vi "AutoCollectBall.vi"(8 "error in (no error)":errorcluster, 10 "PreCollectWait":u32=400, 11 "IsTwoBall?":bool) -> (0 "error out":errorcluster)   [LabVIEW 2013]
uses:
  DoubleSolenoidAction.ctl
  RollerAction.ctl
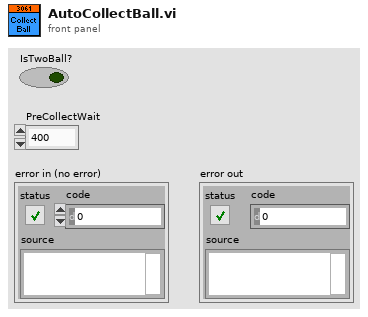
[diagram p1: front panel]
types:
  T1 = typedef "RollerAction.ctl" = enum16{"Init", "Off", "Forward", "Reverse"}
  T2 = typedef "DoubleSolenoidAction.ctl" = enum16{"Init", "Middle", "In", "Out"}
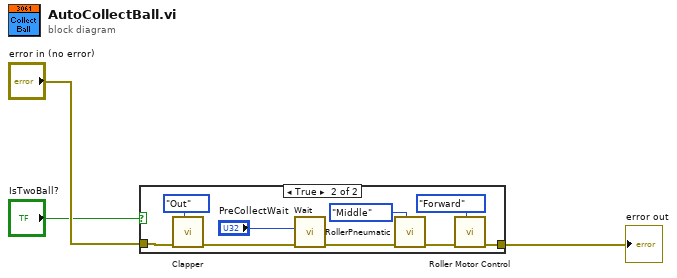
[diagram p0: block diagram]
diagram:
  n1 = case shown="True" "IsTwoBall?" {
    tunnel: [w4 w7] -> w1
    tunnel: "error in (no error)" -> [w4 w8]
    frame False {
    }
    frame True {
      n2 = call "Clapper.vi"("State"=DoubleSolenoidAction."Out", "Error in"=w8) -> ("Error out"=w12:errorcluster)  [unwired: 9 in]
      n3 = call "Wait.vi"("error in"=w12, "milliseconds to wait"="PreCollectWait") -> ("error out"=w10:errorcluster)  [unwired: 9 in]
      n4 = call "RollerPneumatic.vi"("State"=DoubleSolenoidAction."Middle", "Error in"=w10) -> ("Error out"=w13:errorcluster)  [unwired: 9 in]
      n5 = call "Roller Motor Control.vi"("Action"=RollerAction."Forward", "Error in"=w13) -> ("Error out"=w7:errorcluster)  [unwired: 9 in]
    }
  }
  "error out" <- w1
